vi "Generate Diode Map.vi"() -> ()   [LabVIEW 2018]
uses:
  <vilib>/DAQmx/write.llb/DAQmx Write (Analog DBL 1Chan 1Samp).vi
  d3d6812e-0f49-4454-aa36-1c3f2e9fb1ad.vi
  <vilib>/DAQmx/read.llb/DAQmx Read (Analog DBL 1Chan 1Samp).vi
  <vilib>/Analysis/baseanly.llb/Mean (DBL).vi
  <vilib>/DAQmx/create/channels.llb/DAQmx Create Channel (AO-Voltage-Basic).vi
  <vilib>/DAQmx/create/channels.llb/DAQmx Create Channel (AI-Voltage-Basic).vi
  <vilib>/DAQmx/miscellaneous.llb/DAQmx Fill In Error Info.vi
  <vilib>/Analysis/NI_AALBase.lvlib
panel:
  in  "Filename":path=path "polarimeter map.lvm"
  out "XY Graph":cluster{"Y":dbl[], "Y":dbl[]}[](graph)
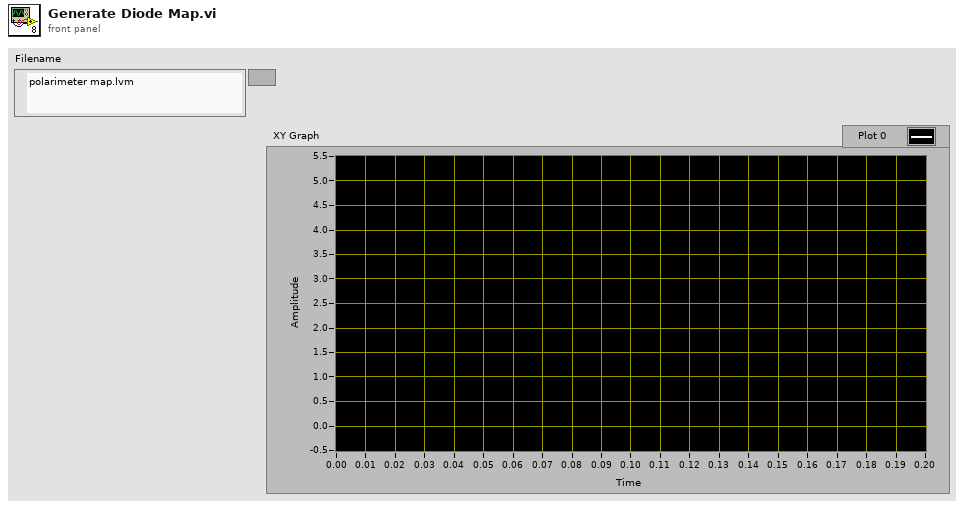
[diagram p1: front panel]
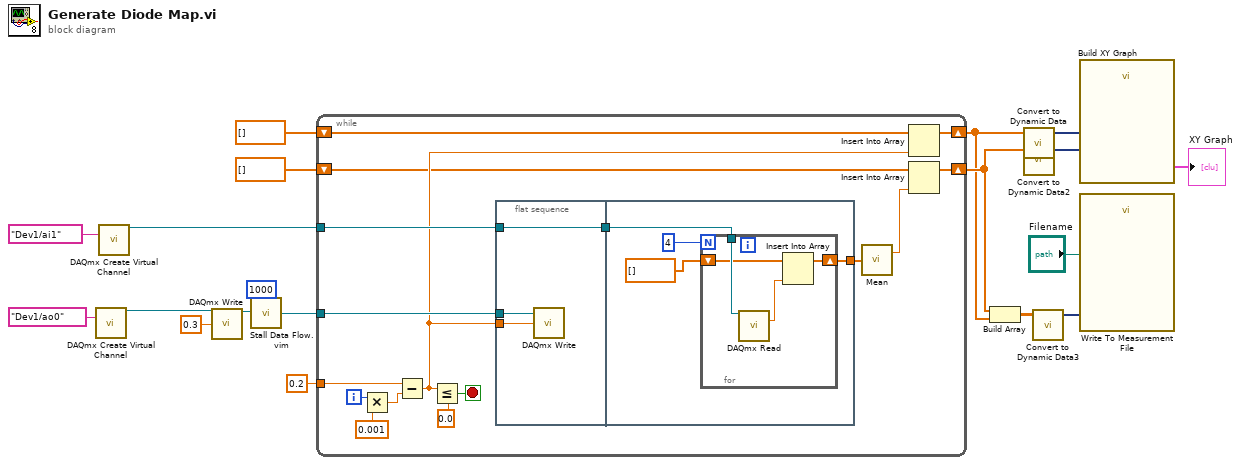
[diagram p0: block diagram]
diagram:
  n1 = call-poly <vilib>:"DAQmx Create Virtual Channel.vi"("physical channels"=tag "Dev1/ao0") -> ("task out"=w15:refnum<k21>)  [unwired: 13 in, 1 out]
  n2 = call-poly <vilib>:"DAQmx Create Virtual Channel.vi"("physical channels"=tag "Dev1/ai1") -> ("task out"=w17:refnum<k21>)  [unwired: 13 in, 1 out]
  n3 = call-poly <vilib>:"DAQmx Write.vi"("task/channels in"=w15, "data"=0.3 ("x")) -> ("task out"=w13:refnum<k21>)  [unwired: 11 in, 2 out]
  n4 = call "Stall Data Flow.vim"("value in"=w13, "milliseconds to wait"=u32 1000) -> ("value out"=w12:refnum<k21>)  [unwired: 1 out]
  n5 = while {
    tunnel: w17 -> [w32]
    shift-right: [w29] -> w5
    shift-left: dbl[] [] -> [w30]
    tunnel: 0.2 ("x") -> [w25]
    tunnel: w12 -> [w24]
    shift-right: [w22] -> w6
    shift-left: dbl[] [] -> [w21]
    i -> [w35]
    stop <- w34 stop-if-true
    n6 = Multiply(x=w35, y=0.001) -> (x*y=w28:dbl)
    n7 = Subtract(x=w25, y=w28) -> (x-y=w23:dbl)
    n8 = Less Or Equal?(x=w23, y=0.0) -> (x <= y?=w34:bool)
    n9 = flat-sequence {
      tunnel: w32 -> [w38]
      tunnel: [w38] -> w26
      tunnel: w23 -> [w37]
      tunnel: w24 -> [w36]
      tunnel: [w39] -> w31
      tunnel: w26 -> [w41]
      frame #0 {
        n10 = call-poly <vilib>:"DAQmx Write.vi"("task/channels in"=w36, "data"=w37) -> ()  [unwired: 11 in, 3 out]
      }
      frame #1 {
        n11 = for {
          N: 4 -> [_]
          tunnel: w41 -> [w46]
          shift-right: [w45] -> w39
          shift-left: dbl[] [] -> [w44]
          n12 = call-poly <vilib>:"DAQmx Read.vi"("task/channels in"=w46) -> ("data"=w43:dbl)  [unwired: 12 in, 2 out]
          n13 = Insert Into Array(array=w44, new element=w43) -> (w45:dbl[])  [unwired: 1 in]
        }
      }
    }
    n14 = call-poly <vilib>:"Mean.vi"("X"=w31) -> ("mean"=w20:dbl)  [unwired: 1 out]
    n15 = Insert Into Array(array=w30, new element=w23) -> (w29:dbl[])  [unwired: 1 in]
    n16 = Insert Into Array(array=w21, new element=w20) -> (w22:dbl[])  [unwired: 1 in]
  }
  n17 = Build Array(w6, w5) -> (w4:dbl[][])
  n18 = call "Convert to Dynamic Data"("Array"=w5) -> ("Dynamic Data Type"=w8:dynamicdata)  [unwired: 3 in]
  n19 = call "Convert to Dynamic Data2"("Array"=w6) -> ("Dynamic Data Type"=w7:dynamicdata)  [unwired: 3 in]
  n20 = call "Convert to Dynamic Data3"("2D Array"=w4) -> ("Dynamic Data Type"=w2:dynamicdata)  [unwired: 3 in]
  n21 = call "Build XY Graph"("Y Input"=w7, "X Input"=w8) -> ("XY Graph"=→"XY Graph":cluster{"X":dbl[], "Y":dbl[]}[])  [unwired: 8 in, 1 out]
  n22 = call "Write To Measurement File"("Signals"=w2, "Filename"="Filename") -> ()  [unwired: 15 in, 3 out]
